vi "test_simple_threshold.vi"() -> ()   [LabVIEW 2009]
doc: "Copyright (C) 2009, Stepan A. Baranov\nweb: http://www.OCTLab.org/\nemail: stepan@baranov.su"
uses:
  OCTLib.dll
panel:
  out "error out":errorcluster
  out "max":dbl
  out "min":dbl
  out "width":i32
  out "height":i32
  in  "Small/Big":bool
  out "loop #":i32
  out "RSM_STAT time":u32
  out "LabView time":u32
  out "RSM_STAT Array":dbl[][](array[numeric])
  out "LabView Array":dbl[][](array[numeric])
  in  "stop":bool
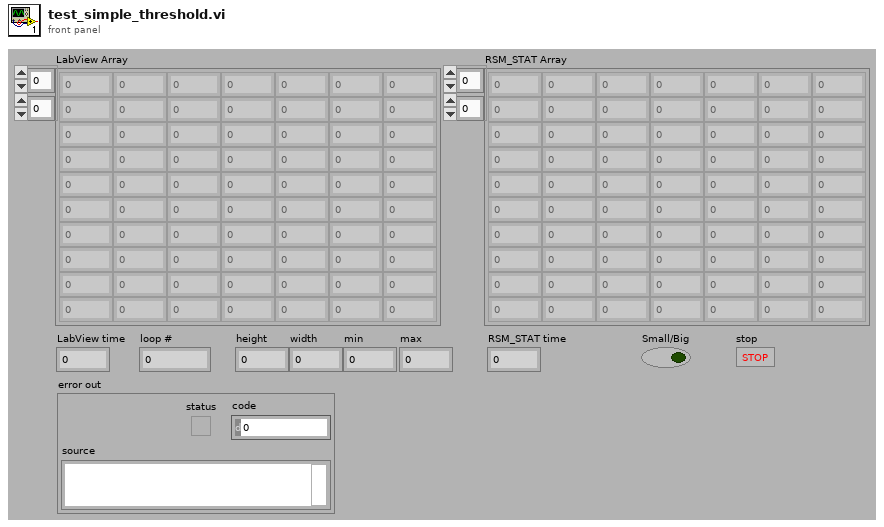
[diagram p1: front panel]
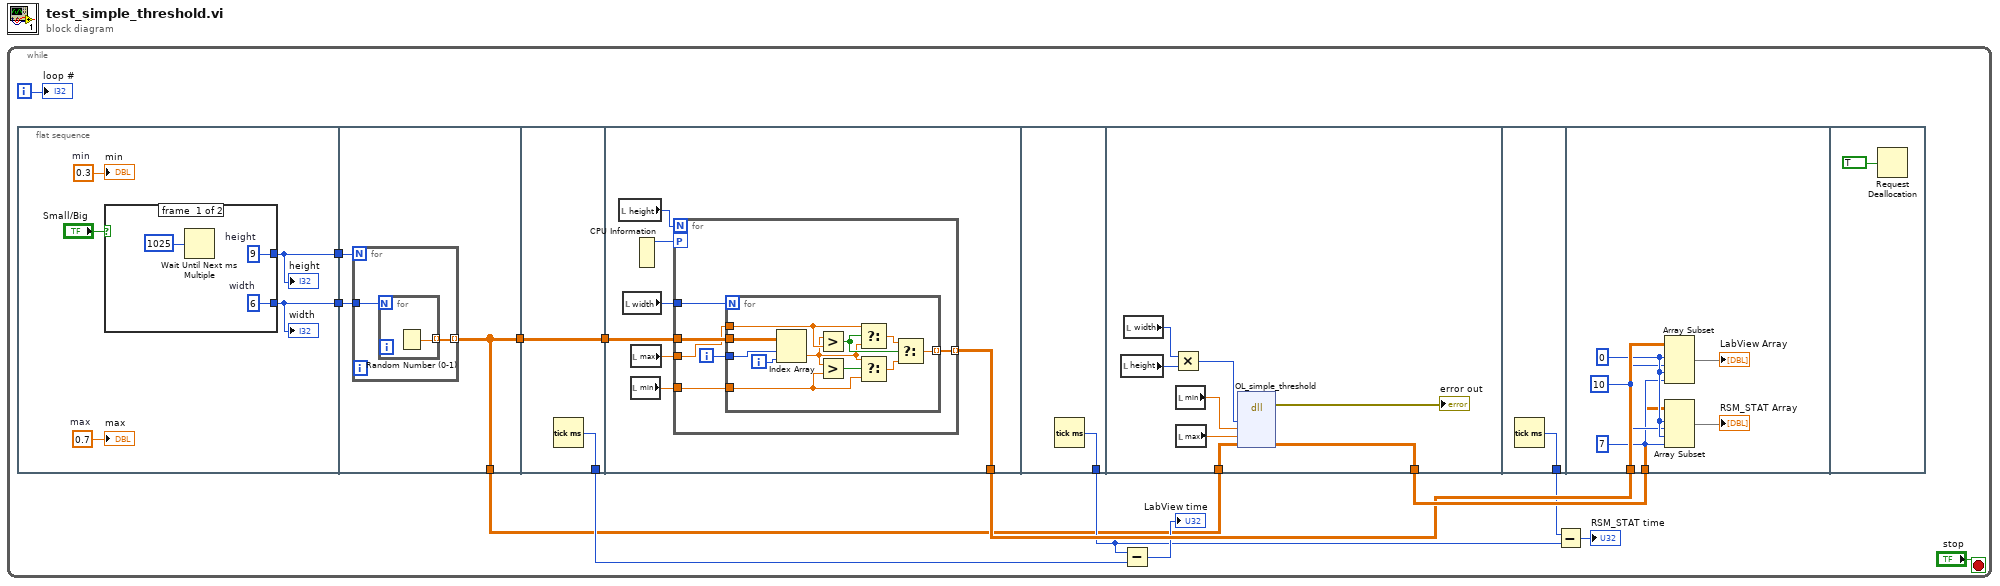
[diagram p0: block diagram]
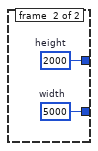
[diagram p2: hidden frame]
diagram:
  n1 = while {
    i -> [w6]
    stop <- "stop" stop-if-true
    n2 = flat-sequence {
      tunnel: [w18] -> w2
      tunnel: [w17] -> w1
      tunnel: [w25] -> w5
      tunnel: [w25] -> w3
      tunnel: w2 -> [w27]
      tunnel: w1 -> [w26]
      tunnel: [w32] -> w11
      tunnel: [w31] -> w4
      tunnel: w3 -> [w31]
      tunnel: [w39] -> w12
      tunnel: w4 -> [w38]
      tunnel: [w57] -> w8
      tunnel: w5 -> [w65]
      tunnel: [w64] -> w13
      tunnel: [w66] -> w9
      tunnel: w13 -> [w67]
      tunnel: w12 -> [w73]
      frame #0 {
        w15 = 0.7  # max
        w16 = 0.3  # min
        n3 = case shown="True" "Small/Big" {
          tunnel: [w21 w24] -> w17
          tunnel: [w22 w23] -> w18
          frame #0 {
            w22 = 6  # width
            w21 = 9  # height
            n4 = Wait Until Next ms Multiple(millisecond multiple=u32 1025) -> ()  [unwired: 1 out]
          }
          frame #1 {
            w23 = 5000  # width
            w24 = 2000  # height
          }
        }
        "height" <- w17
        "width" <- w18
        "min" <- w16
        "max" <- w15
      }
      frame #1 {
        n5 = for {
          N: w26 -> [_]
          tunnel: w27 -> [w29]
          tunnel: [w28] -> w25 mode=indexing
          n6 = for {
            N: w29 -> [_]
            tunnel: [w30] -> w28 mode=indexing
            n7 = Random Number (0-1)() -> (number: 0 to 1=w30:dbl)
          }
        }
      }
      frame #2 {
        n8 = Tick Count (ms)() -> (millisecond timer value=w32:u32)
      }
      frame #3 {
        n9 = local read "height"() -> (w37:i32)
        n10 = local read "width"() -> (w34:i32)
        n11 = local read "max"() -> (w36:dbl)
        n12 = local read "min"() -> (w35:dbl)
        n13 = CPU Information() -> (4:w33:i32)  [unwired: 3 out]
        n14 = for {
          N: w37 -> [_]
          tunnel: w36 -> [w42]
          tunnel: w35 -> [w41]
          tunnel: w34 -> [w40]
          tunnel: w38 -> [w45]
          tunnel: [w43] -> w39 mode=indexing
          workers-P: w33 -> [_]
          i -> [w44]
          n15 = for {
            N: w40 -> [_]
            tunnel: w44 -> [w55]
            tunnel: w42 -> [w53]
            tunnel: w41 -> [w52]
            tunnel: w45 -> [w56]
            tunnel: [w46] -> w43 mode=indexing
            i -> [w54]
            n16 = Index Array(array=w56, index (row)=w55, index (col)=w54) -> (element=w47:dbl)
            n17 = Greater?(x=w47, y=w53) -> (0:w50:bool)
            n18 = Greater?(x=w47, y=w52) -> (0:w51:bool)
            n19 = Select(t=w53, s=w50, f=w47) -> (s? t:f=w49:dbl)
            n20 = Select(t=w47, s=w51, f=w52) -> (s? t:f=w48:dbl)
            n21 = Select(t=w49, s=w50, f=w48) -> (s? t:f=w46:dbl)
          }
        }
      }
      frame #4 {
        n22 = Tick Count (ms)() -> (millisecond timer value=w57:u32)
      }
      frame #5 {
        n23 = local read "height"() -> (w60:i32)
        n24 = local read "width"() -> (w61:i32)
        n25 = Multiply(x=w61, y=w60) -> (x*y=w59:i32)
        n26 = local read "min"() -> (w63:dbl)
        n27 = local read "max"() -> (w62:dbl)
        n28 = dll-call lib="OCTLib.dll" fn="OL_simple_threshold"("size"=w59, "min"=w63, "max"=w62, "data"=w65) -> (error out=→"error out":errorcluster, "data"=w64:dbl[][])  [unwired: 7 in, 1 out]
      }
      frame #6 {
        n29 = Tick Count (ms)() -> (millisecond timer value=w66:u32)
      }
      frame #7 {
        w70 = 10 ("length")
        w69 = 7 ("length")
        w71 = 0 ("index")
        n30 = Array Subset(array=w73, index (row)=w71, length (row)=w70, index (col)=w71, length (col)=w69) -> (→"LabView Array":dbl[][])
        n31 = Array Subset(array=w67, index (row)=w71, length (row)=w70, index (col)=w71, length (col)=w69) -> (→"RSM_STAT Array":dbl[][])
      }
      frame #8 {
        n32 = Request Deallocation(TRUE ("flag")) -> ()
      }
    }
    n33 = Subtract(x=w8, y=w11) -> (x-y=→"LabView time":u32)
    n34 = Subtract(x=w9, y=w8) -> (x-y=→"RSM_STAT time":u32)
    "loop #" <- w6
  }
